vi "LabelPrinter.vi"(4 "Offset (m)":string, 5 "SN":string, 6 "error in (no error)":errorcluster, 7 "Ring Time (ms)":string, 8 "Tube SN":string) -> (0 "error out":errorcluster)   [LabVIEW 2014]
doc: "Pulls in a label template file and prints a label to the Brother label printer in the cal labe with the following:\n\n<B>Label Parameters</B>\nCurrent Date\nSensor SN\nTube SN\nSensor Offset\nTransducer Ring Time"
panel:
  in  "Cancel Button":bool
  in  "Print Label Button":bool
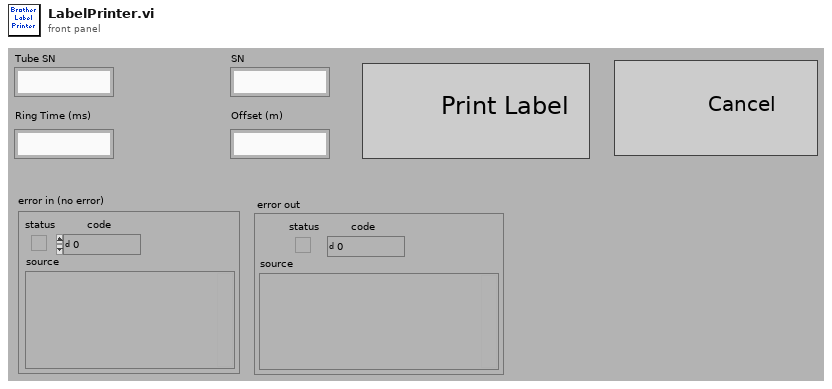
[diagram p1: front panel]
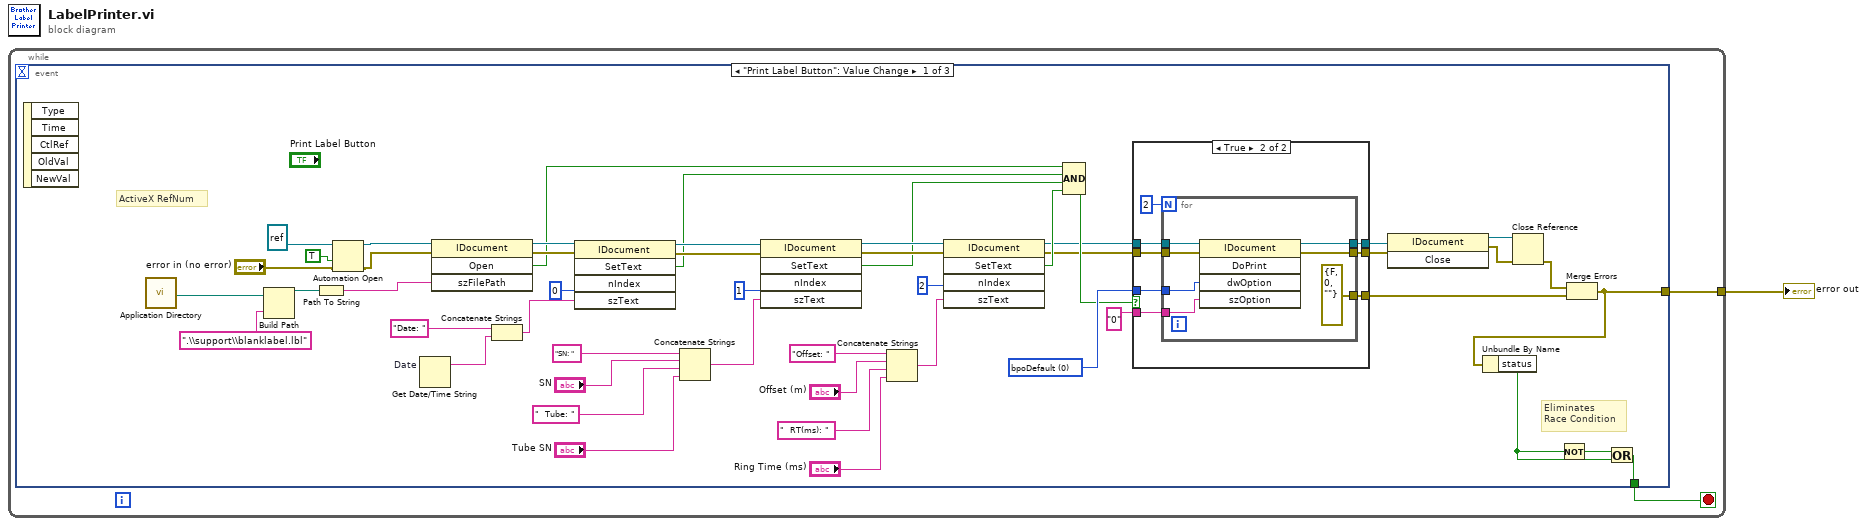
[diagram p0: block diagram]
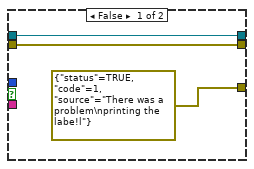
[diagram p2: hidden frame]
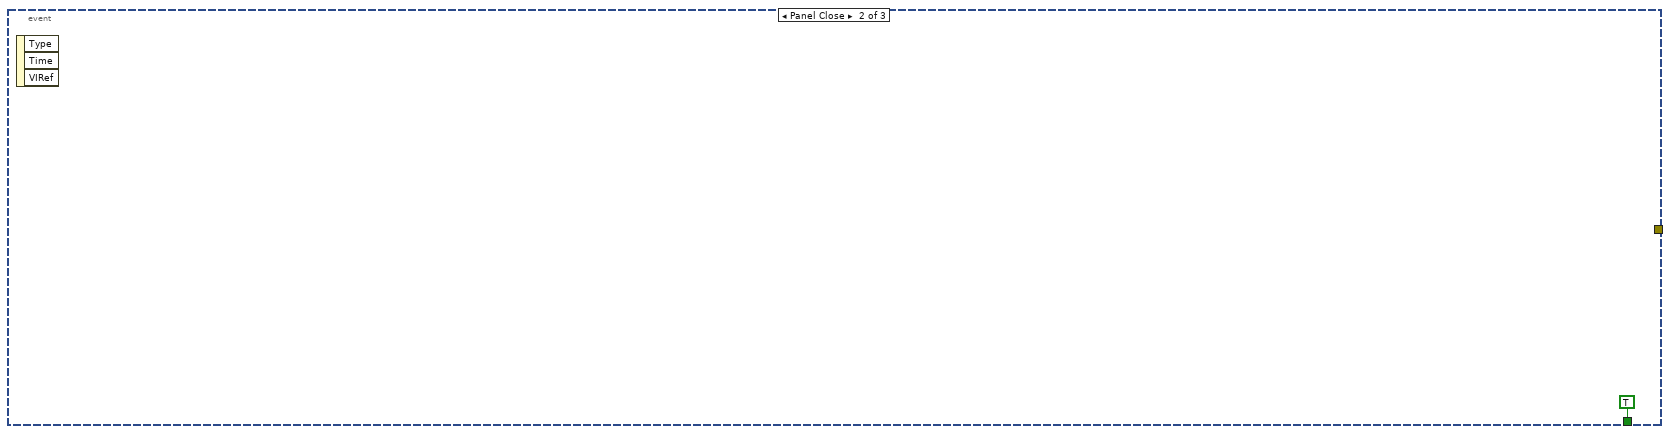
[diagram p3: hidden frame]
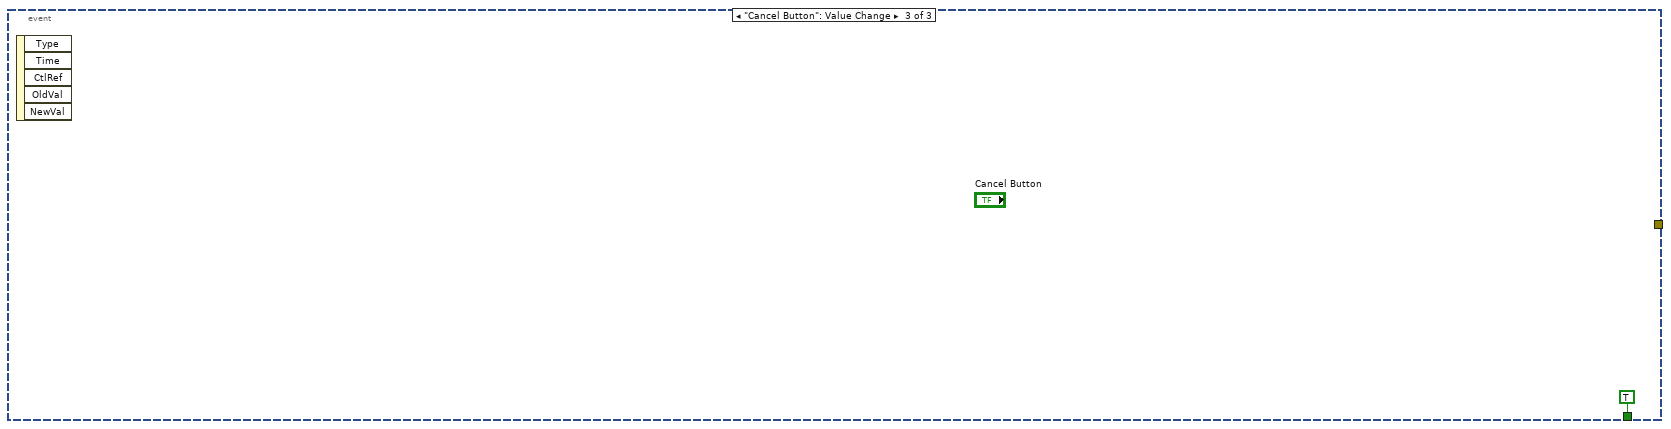
[diagram p4: hidden frame]
diagram:
  n1 = while {
    tunnel: [w3] -> w1
    stop <- w2 stop-if-true
    n2 = event shown="[0] \"Print Label Button\": Value Change" {
      selector: _ -> [_ _ _]
      dyn-events: _ -> [_ _ _]
      timeout: _ -> [_ _ _]
      tunnel: [w15 _ _] -> w3
      tunnel: [w14 TRUE TRUE] -> w2
      event "Print Label Button": Value Change {
        w47 = 0 items=["bpoDefault"=0, "bpoAutoCut"=1, "bpoCutPause"=2, "bpoMirroring"=4, "bpoColor"=8, "bpoStamp"=128, "bpoHalfCut"=512, "bpoMono, bpoNoCut, bpoIdLabel"=268435456] ("dwOption")
        # "Eliminates\nRace Condition"
        # "ActiveX RefNum"
        n3 = event-data() -> ()  [unwired: 1 in, 5 out]
        n4 = call <vilib>:"Application Directory.vi"() -> ("Application Directory"=w11:path)
        n5 = Build Path(base path=w11, name or relative path=".\\support\\blanklabel.lbl") -> (appended path=w9:path)
        n6 = Path To String(path=w9) -> (string=w46:string)
        n7 = Automation Open(error in (no error)="error in (no error)", Automation Refnum=refnum<k7> refnum ("bpac.IDocument"), 9:TRUE ("open new instance (false)")) -> (Automation Refnum=w5:refnum<k7>, error out=w6:errorcluster)  [unwired: 1 in]
        n8 = Get Date/Time String "Date"() -> (date string=w17:string)  [unwired: 3 in, 1 out]
        n9 = invoke class="IDocument" method="Open"(reference=w5, error in=w6, "szFilePath"=w46) -> (reference out=w40:refnum<k7>, error out=w41:errorcluster, "Open"=w32:bool)  [unwired: 1 in, 1 out]
        n10 = Concatenate Strings("Date: ", w17) -> (w16:string)
        n11 = invoke class="IDocument" method="SetText"(reference=w40, error in=w41, "nIndex"=0, "szText"=w16) -> (reference out=w39:refnum<k7>, error out=w38:errorcluster, "SetText"=w31:bool)  [unwired: 1 in, 2 out]
        n12 = Concatenate Strings("SN: ", "SN", "  Tube: ", "Tube SN") -> (w26:string)
        n13 = invoke class="IDocument" method="SetText"(reference=w39, error in=w38, "nIndex"=1, "szText"=w26) -> (reference out=w42:refnum<k7>, error out=w43:errorcluster, "SetText"=w33:bool)  [unwired: 1 in, 2 out]
        n14 = Concatenate Strings("Offset: ", "Offset (m)", "  RT(ms): ", "Ring Time (ms)") -> (w21:string)
        n15 = invoke class="IDocument" method="SetText"(reference=w42, error in=w43, "nIndex"=2, "szText"=w21) -> (reference out=w20:refnum<k7>, error out=w19:errorcluster, "SetText"=w34:bool)  [unwired: 1 in, 2 out]
        n16 = Compound Arithmetic op=AND(w32, w31, w33, w34) -> (w45:bool)
        n17 = case shown="True" w45 {
          tunnel: w47 -> [_ w64]
          tunnel: "0" ("szOption") -> [_ w63]
          tunnel: w19 -> [w54 w62]
          tunnel: w20 -> [w56 w61]
          tunnel: [w56 w60] -> w49
          tunnel: [w54 w59] -> w50
          tunnel: [errorcluster {"status"=TRUE, "code"=1, "source"="There was a problem\nprinting the labe!l"} ("error out") w58] -> w36
          frame False {
          }
          frame True {
            n18 = for {
              N: 2 -> [_]
              tunnel: w64 -> [w71]
              tunnel: w63 -> [w70]
              tunnel: w62 -> [w69]
              tunnel: w61 -> [w68]
              tunnel: [w67] -> w60
              tunnel: [w66] -> w59
              tunnel: [errorcluster {"status"=FALSE, "code"=0, "source"=""} ("error out")] -> w58
              n19 = invoke class="IDocument" method="DoPrint"(reference=w68, error in=w69, "dwOption"=w71, "szOption"=w70) -> (reference out=w67:refnum<k7>, error out=w66:errorcluster)  [unwired: 1 in, 3 out]
            }
          }
        }
        n20 = invoke class="IDocument" method="Close"(reference=w49, error in=w50) -> (reference out=w52:refnum<k7>, error out=w51:errorcluster)  [unwired: 1 in, 1 out]
        n21 = Close Reference(reference=w52, error in (no error)=w51) -> (error out=w35:errorcluster)
        n22 = Merge Errors(w35, w36) -> (w15:errorcluster)
        n23 = Unbundle By Name(w15) -> ("status"=w12:bool)
        n24 = Not(x=w12) -> (.not. x?=w13:bool)
        n25 = Or(x=w13, y=w12) -> (x .or. y?=w14:bool)
      }
      event Panel Close {
        n26 = event-data() -> ()  [unwired: 1 in, 3 out]
      }
      event "Cancel Button": Value Change {
        n27 = event-data() -> ()  [unwired: 1 in, 5 out]
      }
    }
  }
  "error out" <- w1
